vi "Write.vi"(8 "error in (no error)":errorcluster, 10 "Modbus-Reg":u16[](array[numeric]), 11 "object in":refnum<class "Pressure-Transducer.lvclass">) -> (0 "error out":errorcluster, 3 "object out":refnum<class "Pressure-Transducer.lvclass">)   [LabVIEW 2021, in "Pressure-Transducer.lvclass"]
doc: "Write modbus reg"
uses:
  Pressure-Transducer.lvclass
  Modbus-Instr_class/Modbus-Instr.lvclass
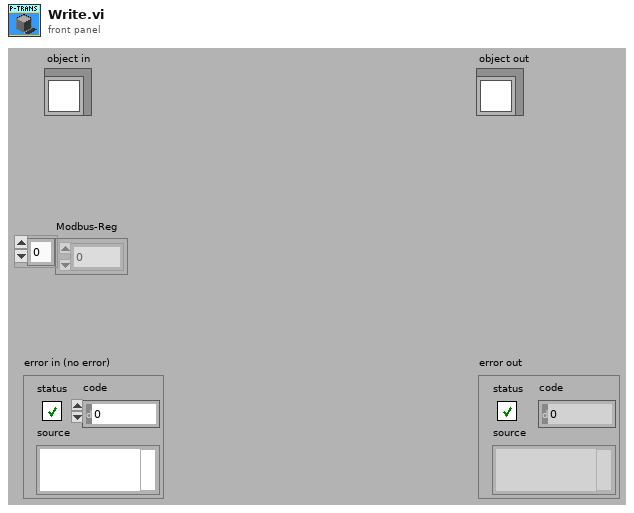
[diagram p1: front panel]
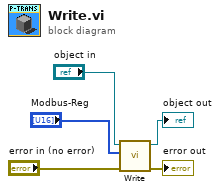
[diagram p0: block diagram]
diagram:
  n1 = call-parent "Write.vi"("error in (no error)"="error in (no error)", "Modbus-Reg"="Modbus-Reg", "object in"="object in") -> ("error out"=→"error out":errorcluster, "object out"=→"object out":refnum<class "Pressure-Transducer.lvclass">)  [unwired: 7 in]
